vi "DAQ.TimedLoop.vi"(8 "error in (no error)":errorcluster, 10 "Event Cluster":T1, 11 "Instrument.DAQ in":refnum<class "Instrument.DAQ.lvclass">) -> (0 "error out":errorcluster, 3 "Instrument.DAQ out":refnum<class "Instrument.DAQ.lvclass">)   [LabVIEW 2019, in "Instrument.DAQ.lvclass"]
uses:
  Instrument.DAQ.lvclass
  <vilib>/JKI/JKI SMO/SMO/Typedefs/Protected Events.ctl
  <vilib>/JKI/JKI SMO/SMO/Typedefs/StopProcessEventData--Cluster.ctl
  <vilib>/JKI/JKI SMO/SMO/Typedefs/AbortProcessEventData--Cluster.ctl
  <vilib>/JKI/JKI SMO/SMO/Typedefs/SMO Dependency Event--Cluster.ctl
  <vilib>/JKI/JKI SMO/SMO/Typedefs/SMO Dependency Event--Enum.ctl
  Typedefs/PrivateEvents--Cluster.ctl
  Typedefs/PrivateEvents--DAQ.setAOconfig.ctl
  Typedefs/DAQ.Config.AO--Cluster--Array.ctl
  Typedefs/DAQ.Config.AO--Cluster.ctl
  Typedefs/DAQ.Config.AO.Range--enum.ctl
  Typedefs/DAQ.Type--enum.ctl
  Typedefs/PrivateEvents--DAQ.setAIconfig.ctl
  Typedefs/DAQ.Config.AI--Cluster--Array.ctl
  Typedefs/DAQ.Config.AI--Cluster.ctl
  Typedefs/DAQ.Config.AI.Coupling--enum.ctl
  Typedefs/DAQ.Config.AI.Range--enum.ctl
  Typedefs/Simulation Mode--enum.ctl
  Typedefs/PrivateEvents--DAQ.setAO.ctl
  Typedefs/AO.Channel--Cluster--Array.ctl
  Typedefs/AO.Channel--Cluster.ctl
  Typedefs/AO.Channel.Function--Enum.ctl
  Typedefs/PrivateEvents--DAQ.setREF.ctl
  Typedefs/REF.Channel--Cluster--Array.ctl
  Typedefs/REF.Channel--Cluster.ctl
  Typedefs/PrivateEvents--DAQ.setSampling.ctl
  Typedefs/DAQ.Sampling.Sampling--Cluster.ctl
  Typedefs/DAQ.Sampling.Sample Mode--Ring.ctl
  Typedefs/PrivateEvents--DAQ.setState.ctl
  Typedefs/Set State-enum.ctl
  Typedefs/PrivateEvents--DAQ.setInputGain.ctl
  Typedefs/PrivateEvents--DAQ.setSweep.ctl
  Typedefs/Sweep.Configuration--Cluster.ctl
  Typedefs/Sweep.Channel--Cluster--Array.ctl
  Typedefs/Sweep.Channel--Cluster.ctl
  Typedefs/Sweep.Pattern--Enum.ctl
  Typedefs/PrivateEvents--DAQ.measureOffset.ctl
  Typedefs/PrivateEvents--DAQ.zeroOffset.ctl
  Typedefs/PrivateEvents--DAQ.setPreFilter.ctl
  Typedefs/Configuration.Prefilter--Cluster.ctl
  Typedefs/PrivateEvents--DAQ.autoConfigureDAQ.ctl
  Typedefs/PrivateEvents--DAQ.setCalibration.ctl
  Typedefs/PrivateEvents--DAQ.setAI.ctl
  Typedefs/AI.Channel--Cluster--Array.ctl
  Typedefs/AI.Channel--Cluster.ctl
  Typedefs/PrivateEvents--DAQ.zeroPhase.ctl
  Typedefs/PrivateEvents--DAQ.setLimitAmplitude.ctl
  Typedefs/Configuration.LimitAmplitude--Cluster.ctl
  Typedefs/PrivateEvents--DAQ.setLinkFrequencies.ctl
  Typedefs/Configuration.LinkFrequencies--Cluster.ctl
  <vilib>/Platform/TimedLoop/XDataNode/wakeup.ctl
  <vilib>/Platform/TimedLoop/XDataNode/XDNodeRunTimeDep.lvlib
  <vilib>/Platform/TimedLoop/XDataNode/nitl_modes.ctl
  <vilib>/Platform/TimedLoop/XDataNode/timing_clust.ctl
  <vilib>/platform/TimedLoop/XDataNode/XDataNode.xnode
  <vilib>/JKI/JKI SMO/SMO/SMO.lvclass
  C:/Program Files (x86)/National Instruments/LabVIEW 2019/vi.lib/JKI/JKI SMO/SMO/SMO.lvclass
panel:
  out "Lockin":u32
  out "AO/AI":u32
  out "generate":u32
  # "!!!!!!!!!!!!!!!!!!!!!!!!!!!!!!!!!!!!!!!!!!!!!!!!!!!!!!!!!!!!!!!!!!!!!!!!\nTHIS IS AN EXPERIMENTAL BLOCKING CALL TO:\nGenerate\nRead/Write\nDSP\nIt should listen to events that change AO or REF Channels.\nInside there is a timed loop that will not stop unless it receives events for Set State = stop; SMO Stop; or SMO error\n!!!!!!!!!!!!!!!!!!!!!!!!!!!!!!!!!!!!!!!!!!!!!!!!!!!!!!!!!!!!!!!!!!!!!"
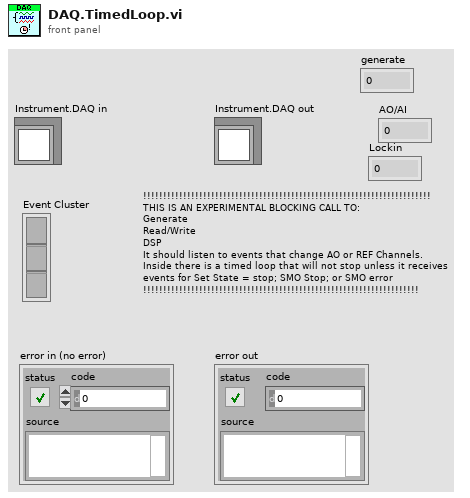
[diagram p1: front panel]
types:
  T1 = cluster{"SMO":refnum<event-registration>, "LockinDAQ":refnum<event-registration>, "DAQmx":refnum<event-registration>}
  T2 = typedef "Instrument.DAQ.lvclass/Set State-enum.ctl" = enum16{"start", "stop", "reset", "start sweep", "stop sweep"}
  T3 = typedef "XDNodeRunTimeDep.lvlib/timing_clust.ctl" = cluster{"Expected End [f-1]":u64, "Actual End [f-1]":u64, "Finished Late? [f-1]":bool, "Expected End [i-1]":u64, "Actual End [i-1]":u64, "Finished Late? [i-1]":bool, "Expected Start [i]":u64, "Actual Start [i]":u64, "Expected Start [f]":u64, "Actual Start [f]":u64, "Source Name":string, "Structure Name":string, "Period":i64, "Deadline":i64, "Offset":i64, "Start":i64, "Priority":i32, "Timeout":i32, "Mode":T4, "Wakeup Reason":T5, "Error":errorcluster, "Source Type":string, "Secondary Source Type":string, "Global End Time":u64, "Global Start Time":u64, "Frame Duration":u64, "Iteration Duration":u64, "Assigned CPU":i32, "I/O Scan Engine Mode":u32}
  T4 = typedef "XDNodeRunTimeDep.lvlib/nitl_modes.ctl" = enum32{"No Change", "Process missed periods, maintain original phase", "Discard missed periods, maintain original phase", "Process missed periods, ignore original phase", "Discard missed periods, ignore original phase"}
  T5 = typedef "XDNodeRunTimeDep.lvlib/wakeup.ctl" = enum32{"Normal", "Aborted", "Asynchronous wakeup", "Timing source error", "Timed loop error", "Timeout"}
  T6 = typedef "SMO.lvclass/Protected Events.ctl" = cluster{"StopProcesses":refnum<user-event>, "AbortProcesses":refnum<user-event>, "Config Changed":refnum<user-event>, "Dependency":refnum<user-event>}
  T7 = typedef "Instrument.DAQ.lvclass/PrivateEvents--Cluster.ctl" = cluster{"setAOconfig":refnum<user-event>, "setAIconfig":refnum<user-event>, "setAO":refnum<user-event>, "setREF":refnum<user-event>, "setSampling":refnum<user-event>, "setState":refnum<user-event>, "setInputGain":refnum<user-event>, "setOutputGain":refnum<user-event>, "setSweep":refnum<user-event>, "measureOffset":refnum<user-event>, "zeroOffset":refnum<user-event>, "setPreFilter":refnum<user-event>, "autoConfigureDAQ":refnum<user-event>, "setCalibration":refnum<user-event>, "setAI":refnum<user-event>, "zeroPhase":refnum<user-event>, "setLimitAmplitude":refnum<user-event>, "setLinkFrequencies":refnum<user-event>}
  T8 = typedef "Instrument.DAQ.lvclass/Results--Cluster.ctl" = cluster{"Time Stamp":timestamp, "Results (Dictionary)":cluster{"key":string, "value":dbl}[]}
  T9 = typedef "Instrument.DAQ.lvclass/AO.Channel--Cluster--Array.ctl" = T10[]
  T10 = typedef "Instrument.DAQ.lvclass/AO.Channel--Cluster.ctl" = cluster{"Enable?":bool, "Channel":i32, "Amplitude":dbl, "Offset":dbl, "Frequency":dbl, "Phase":dbl, "Function":T11, "Sweeping?":bool}
  T11 = typedef "Instrument.DAQ.lvclass/AO.Channel.Function--Enum.ctl" = enum16{"Sine", "Triangle", "Square"}
  T12 = typedef "Instrument.DAQ.lvclass/REF.Channel--Cluster--Array.ctl" = T13[]
  T13 = typedef "Instrument.DAQ.lvclass/REF.Channel--Cluster.ctl" = cluster{"Enable?":bool, "Channel":i32, "Frequency":dbl, "Phase":dbl, "TC":dbl, "Roll-Off":i32}
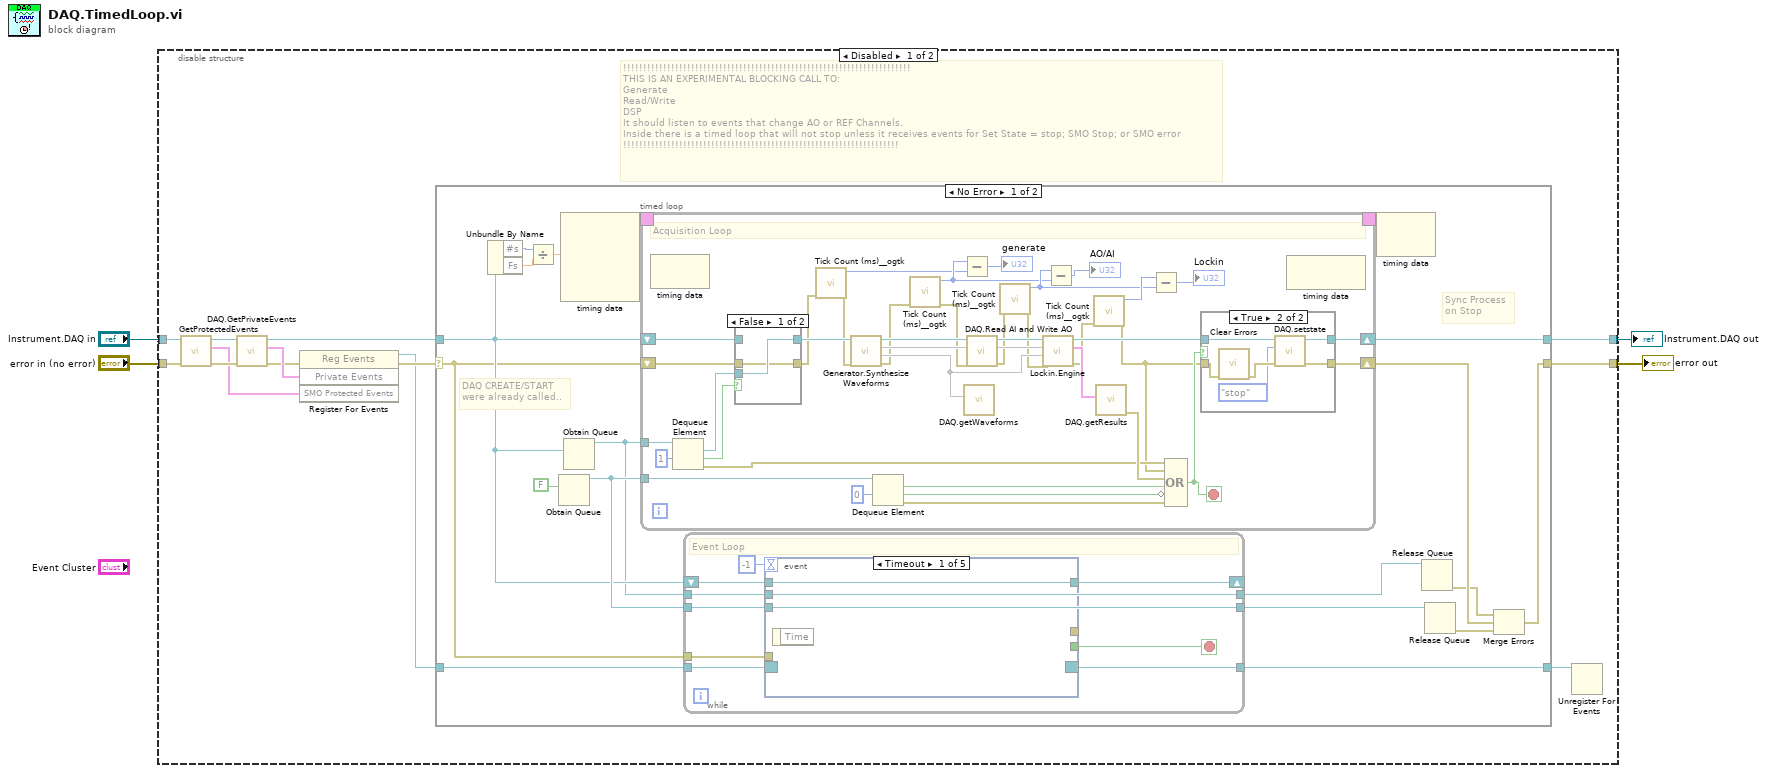
[diagram p0: block diagram]
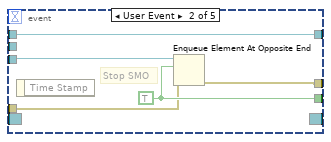
[diagram p4: hidden frame]
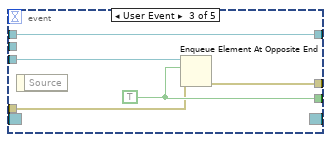
[diagram p5: hidden frame]
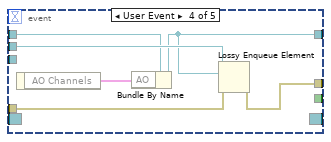
[diagram p6: hidden frame]
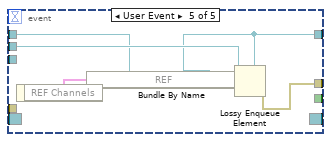
[diagram p7: hidden frame]
diagram:
  n1 = disable-structure shown="Disabled" {
    disable-tunnel: "Instrument.DAQ in" -> [w15 w134]
    disable-tunnel: [w14 w134] -> w3
    disable-tunnel: "error in (no error)" -> [w13 _]
    disable-tunnel: [w5 _] -> w1
    frame Disabled {
      # "!!!!!!!!!!!!!!!!!!!!!!!!!!!!!!!!!!!!!!!!!!!!!!!!!!!!!!!!!!!!!!!!!!!!!!!!\nTHIS IS AN EXPERIMENTAL BLOCKING CALL TO:\nGenerate\nRead/Write\nDSP\nIt should listen to events that change AO or REF Channels.\nInside there is a timed loop that will not stop unless it receives events for Set State = stop; SMO Stop; or SMO error\n!!!!!!!!!!!!!!!!!!!!!!!!!!!!!!!!!!!!!!!!!!!!!!!!!!!!!!!!!!!!!!!!!!!!!"
      n2 = call <vilib>:"GetProtectedEvents.vi"("error in (no error)"=w13, "SMO"=w15) -> ("error out"=w11:errorcluster, "SMO Protected Events"=w10:T6, "SMO out"=w12:refnum<class "Instrument.DAQ.lvclass">)  [unwired: 7 in]
      n3 = call "DAQ.GetPrivateEvents.vi"("error in (no error)"=w11, "Instrument.DAQ"=w12) -> ("error out"=w7:errorcluster, "Private Events"=w9:T7, "Instrument.DAQ out"=w8:refnum<class "Instrument.DAQ.lvclass">)  [unwired: 7 in]
      n4 = register-events(error in=w7, w9, w10) -> (reference out=w6:refnum<event-registration>, error out=w17:errorcluster)  [unwired: 1 in]
      n5 = case shown="No Error" w17 {
        selector: w17 -> [w22 w131]
        tunnel: w8 -> [w23 w132]
        tunnel: w6 -> [w34 w133]
        tunnel: [w28 w131] -> w5
        tunnel: [w33 w133] -> w16
        tunnel: [w19 w132] -> w14
        frame No Error {
          # "DAQ CREATE/START\nwere already called.."
          # "Sync Process\non Stop"
          n6 = Unbundle By Name(w23) -> ("#s"=w27:i32, "Fs"=w25:dbl)
          n7 = Divide(x=w27, y=w25) -> (x/y=w26:dbl)
          n8 = Obtain Queue(element data type=FALSE) -> (queue out=w31:refnum<queue>)  [unwired: 4 in, 2 out]
          n9 = node-c288(w26) -> (w36:T3)  [unwired: 3 in]
          n10 = Obtain Queue(element data type=w23) -> (queue out=w18:refnum<queue>)  [unwired: 4 in, 2 out]
          n11 = timed-loop {
            timing: w36 -> [_]
            timing-out: [_] -> w35
            tunnel: w31 -> [w79]
            shift-right: [w53] -> w19
            shift-left: w23 -> [w58]
            shift-right: [w52] -> w24
            shift-left: w22 -> [w57]
            tunnel: w18 -> [w63]
            stop <- w55 stop-if-true
            # "Acquisition Loop"
            n12 = node-c288() -> ()  [unwired: 1 in, 1 out]
            n13 = Dequeue Element(queue=w63, timeout in ms (-1)=1) -> (element=w60:refnum<class "Instrument.DAQ.lvclass">, timed out?=w61:bool, error out=w56:errorcluster)  [unwired: 1 in, 1 out]
            n14 = case shown="False" w61 {
              tunnel: w60 -> [w89 _]
              tunnel: [w89 w91] -> w59
              tunnel: w58 -> [_ w91]
              tunnel: w57 -> [w88 w90]
              tunnel: [w88 w90] -> w51
              frame False {
              }
              frame True {
              }
            }
            n15 = call <userlib>:"Tick Count (ms)__ogtk.vi"("error in (no error)"=w51) -> ("error out"=w50:errorcluster, "millisecond timer value"=w40:u32)  [unwired: 9 in]
            n16 = call "Generator.Synthesize Waveforms.vi"("error in (no error)"=w50, "Instrument.DAQ"=w59) -> ("error out"=w49:errorcluster, 1:w68, 2:w73, "Instrument.DAQ"=w74:refnum<class "Instrument.DAQ.lvclass">)  [unwired: 6 in]
            n17 = Dequeue Element(queue=w79, timeout in ms (-1)=0) -> (element=w77:bool, timed out?=w76:bool, error out=w75:errorcluster)  [unwired: 1 in, 1 out]
            n18 = call <userlib>:"Tick Count (ms)__ogtk.vi"("error in (no error)"=w49) -> ("error out"=w48:errorcluster, "millisecond timer value"=w41:u32)  [unwired: 9 in]
            n19 = Subtract(x=w41, y=w40) -> (x-y=→"generate":u32)
            n20 = call "DAQ.getWaveforms.vi"("Waveforms"=w68) -> ("error out"=w72:errorcluster, "Instrument.DAQ"=w71:refnum<class "Instrument.DAQ.lvclass">)  [unwired: 9 in]
            n21 = call "DAQ.Read AI and Write AO.vi"("error in (no error)"=w48, 10:w73, "Instrument.DAQ in"=w74) -> ("error out"=w47:errorcluster, 2:w70, "Instrument.DAQ out"=w69:refnum<class "Instrument.DAQ.lvclass">)  [unwired: 6 in]
            n22 = call <userlib>:"Tick Count (ms)__ogtk.vi"("error in (no error)"=w47) -> ("error out"=w46:errorcluster, "millisecond timer value"=w42:u32)  [unwired: 9 in]
            n23 = call "Lockin.Engine.vi"("error in (no error)"=w46, 9:w68, 10:w70, "Instrument.DAQ"=w69) -> ("error out"=w45:errorcluster, "<Results> (X,Y,R,Theta,Mean)"=w65:T8, "Instrument.DAQ out"=w54:refnum<class "Instrument.DAQ.lvclass">)  [unwired: 4 in, 1 out]
            n24 = Subtract(x=w42, y=w41) -> (x-y=→"AO/AI":u32)
            n25 = call <userlib>:"Tick Count (ms)__ogtk.vi"("error in (no error)"=w45) -> ("error out"=w44:errorcluster, "millisecond timer value"=w43:u32)  [unwired: 9 in]
            n26 = call "DAQ.getResults.vi"("Results"=w65) -> ("error out"=w64:errorcluster, "error in (no error)"=w67:errorcluster, "Instrument.DAQ"=w66:refnum<class "Instrument.DAQ.lvclass">)  [unwired: 7 in, 1 out]
            n27 = Subtract(x=w43, y=w42) -> (x-y=→"Lockin":u32)
            n28 = Compound Arithmetic op=OR(w56, w44, w64, w77, invert w76, w75) -> (w55:bool)
            n29 = case shown="True" w55 {
              tunnel: w54 -> [w80 w87]
              tunnel: [w80 w86] -> w53
              tunnel: [w81 w85] -> w52
              tunnel: w44 -> [w81 w83]
              frame False {
              }
              frame True {
                n30 = call <vilib>:"Clear Errors.vi"("error in (no error)"=w83) -> ("error out"=w84:errorcluster)  [unwired: 5 in, 1 out]
                n31 = call "DAQ.setstate.vi"("error in (no error)"=w84, "setState"=Set_State-enum."stop", "Instrument.DAQ"=w87) -> ("error out"=w85:errorcluster, "Instrument.DAQ out"=w86:refnum<class "Instrument.DAQ.lvclass">)  [unwired: 7 in]
              }
            }
            n32 = node-c288() -> ()  [unwired: 1 in, 1 out]
          }
          n33 = while {
            tunnel: w34 -> [w104]
            tunnel: [w103] -> w33
            shift-right: [w100] -> _
            shift-left: w23 -> [w101]
            tunnel: w22 -> [w99]
            tunnel: w18 -> [w98]
            tunnel: [w98] -> w21
            tunnel: w31 -> [w97]
            tunnel: [w97] -> w30
            stop <- w102 stop-if-true
            # "Event Loop"
            n34 = event shown="[0] Timeout" {
              selector: w104 -> [_ _ _ _ _]
              dyn-events: [_ _ _ _ _] -> w103
              timeout: -1 -> [_ _ _ _ _]
              tunnel: [_ w110 w113 _ _] -> w102
              tunnel: w97 -> [_ w111 w116 _ _]
              tunnel: [_ w107 w115 w121 w126] -> _
              tunnel: w101 -> [w106 w109 w114 w120 w125]
              tunnel: [w106 w109 w114 w118 w123] -> w100
              tunnel: w99 -> [_ w108 w112 w117 w129]
              tunnel: w98 -> [_ _ _ w122 w128]
              event Timeout {
                n35 = event-data() -> ()  [unwired: 1 in, 1 out]
              }
              event User Event {
                w110 = TRUE
                # "Stop SMO"
                n36 = event-data() -> ()  [unwired: 1 in, 1 out]
                n37 = Enqueue Element At Opposite End(queue=w111, element=w110, error in (no error)=w108) -> (error out=w107:errorcluster)  [unwired: 1 in, 2 out]
              }
              event User Event {
                w113 = TRUE
                n38 = event-data() -> ()  [unwired: 1 in, 1 out]
                n39 = Enqueue Element At Opposite End(queue=w116, element=w113, error in (no error)=w112) -> (error out=w115:errorcluster)  [unwired: 1 in, 2 out]
              }
              event User Event {
                n40 = event-data() -> ("AO Channels"=w119:T9)  [unwired: 1 in]
                n41 = Bundle By Name(cluster=w120, "AO"=w119) -> (w118:refnum<class "Instrument.DAQ.lvclass">)
                n42 = Lossy Enqueue Element(queue=w122, element=w118, error in (no error)=w117) -> (error out=w121:errorcluster)  [unwired: 3 out]
              }
              event User Event {
                n43 = event-data() -> ("REF Channels"=w124:T12)  [unwired: 1 in]
                n44 = Bundle By Name(cluster=w125, "REF"=w124) -> (w123:refnum<class "Instrument.DAQ.lvclass">)
                n45 = Lossy Enqueue Element(queue=w128, element=w123) -> (error in (no error)=w127:errorcluster, error out=w126:errorcluster)  [unwired: 3 out]
              }
            }
          }
          n46 = node-c288(w35) -> ()  [unwired: 1 out]
          n47 = Release Queue(queue=w21) -> (error out=w20:errorcluster)  [unwired: 2 in, 2 out]
          n48 = Release Queue(queue=w30) -> (error out=w29:errorcluster)  [unwired: 2 in, 2 out]
          n49 = Merge Errors(w20, w24, w29) -> (w28:errorcluster)
        }
        frame Error {
        }
      }
      n50 = Unregister For Events(event registration refnum=w16) -> ()  [unwired: 1 in, 1 out]
    }
    frame Enabled {
    }
  }
  "Instrument.DAQ out" <- w3
  "error out" <- w1
